vi "WF_Load_single_file_with_params.vi"(5 "Record#_START":i32, 8 "N of Record":i32, 9 "Record# STOP":i32, 10 "Enable limit = True":bool, 11 "WF_FILE_IN":path) -> (1 "Sampling rate":dbl, 2 "Record#":i32, 3 "Waveform":waveform(dbl), 4 "File_duration(s)":dbl)   [LabVIEW 2017]
uses:
  <vilib>/Waveform/WDTFileIO.llb/Read Waveform from File.vi
  <vilib>/Waveform/WDTOps.llb/WDT Append Waveforms DBL.vi
panel:
  out "Waveform Graph":waveform(dbl)(graph)
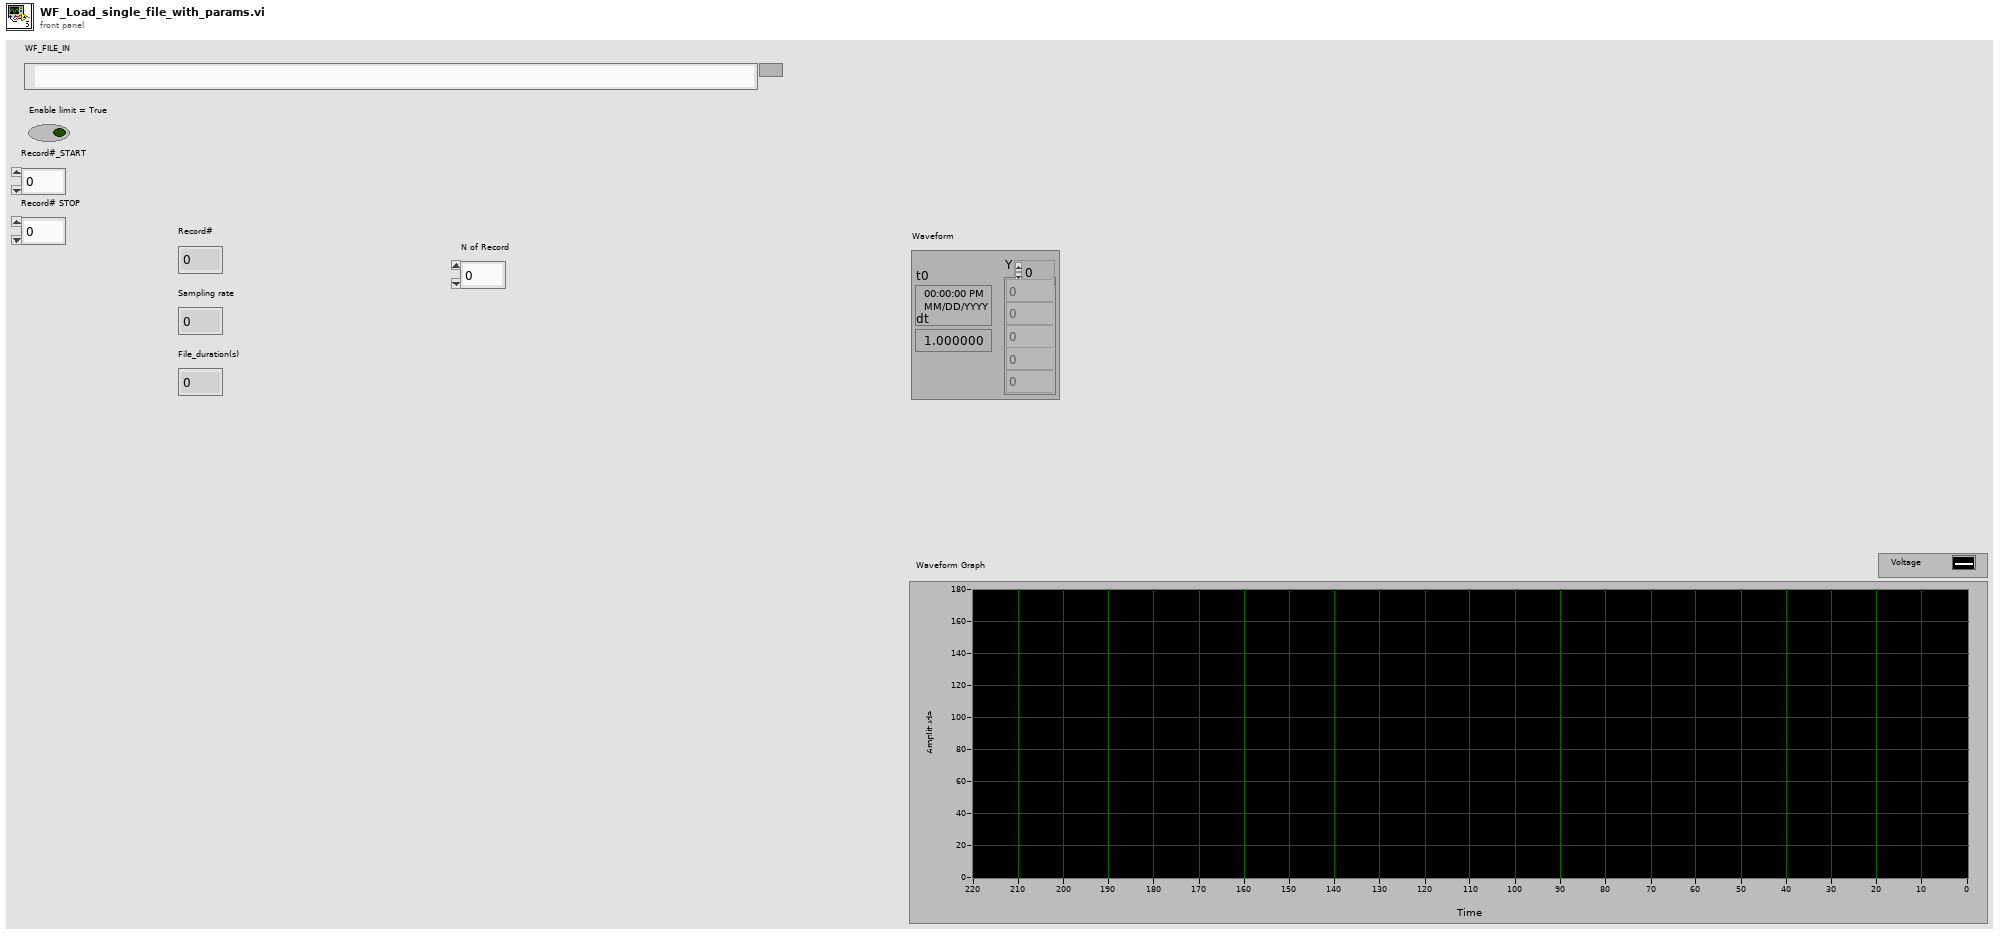
[diagram p1: front panel]
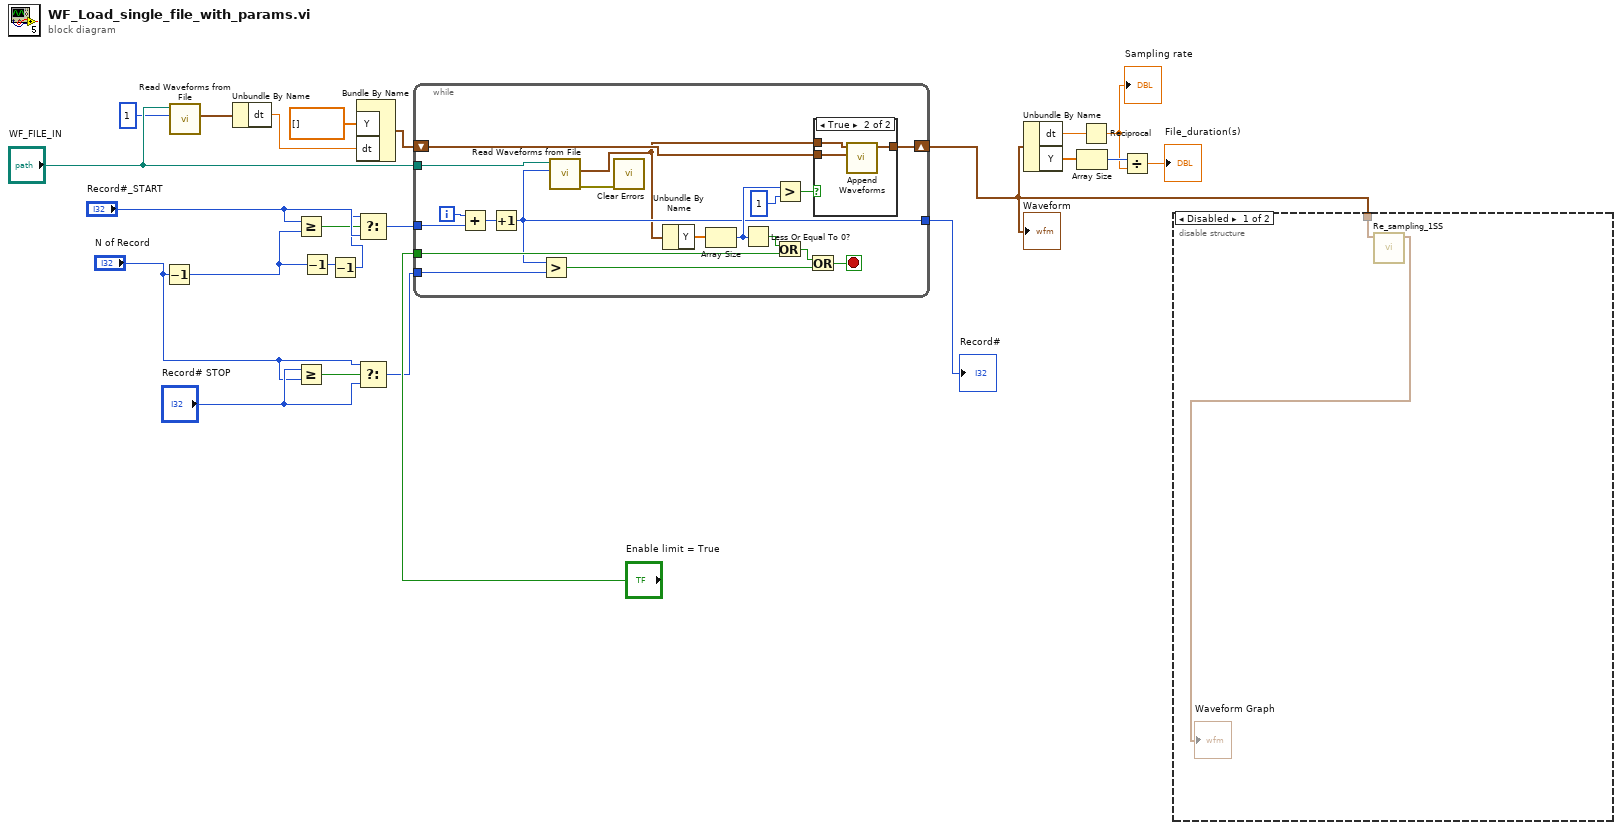
[diagram p0: block diagram]
diagram:
  n1 = Decrement(x="N of Record") -> (x-1=w5:i32)
  n2 = call-poly <vilib>:"Read Waveforms from File.vi"("offset (records:0)"=1, "file path (dialog if empty)"="WF_FILE_IN") -> ("first waveform in record"=w13:waveform(dbl))  [unwired: 4 in, 3 out]
  n3 = Unbundle By Name(w13) -> ("dt"=w16:dbl)
  n4 = Greater Or Equal?(x="Record#_START", y=w5) -> (x >= y?=w9:bool)
  n5 = Greater Or Equal?(x="Record# STOP", y="N of Record") -> (x >= y?=w7:bool)
  n6 = Decrement(x=w5) -> (x-1=w4:i32)
  n7 = Decrement(x=w4) -> (x-1=w3:i32)
  n8 = Bundle By Name("Y"=dbl[] [], "dt"=w16) -> (w17:waveform(dbl))  [unwired: 1 in]
  n9 = Select(t=w3, s=w9, f="Record#_START") -> (s? t:f=w10:i32)
  n10 = Select(t="N of Record", s=w7, f="Record# STOP") -> (s? t:f=w6:i32)
  n11 = while {
    shift-right: [w43] -> w1
    shift-left: w17 -> [w39]
    tunnel: "WF_FILE_IN" -> [w42]
    tunnel: "Enable limit = True" -> [w32]
    tunnel: [w30] -> w20
    tunnel: w10 -> [w31]
    tunnel: w6 -> [w29]
    i -> [w34]
    stop <- w26 stop-if-true
    n12 = Add(x=w34, y=w31) -> (x+y=w33:i32)
    n13 = Increment(x=w33) -> (x+1=w30:i32)
    n14 = Greater?(x=w30, y=w29) -> (0:w28:bool)
    n15 = call-poly <vilib>:"Read Waveforms from File.vi"("offset (records:0)"=w30, "file path (dialog if empty)"=w42) -> ("error out"=w40:errorcluster, "first waveform in record"=w25:waveform(dbl))  [unwired: 4 in, 2 out]
    n16 = call <vilib>:"Clear Errors.vi"("error in (no error)"=w40) -> ()  [unwired: 5 in, 2 out]
    n17 = Unbundle By Name(w25) -> ("Y"=w41:dbl[])
    n18 = Array Size(array=w41) -> (size(s)=w36:i32)
    n19 = Less Or Equal To 0?(x=w36) -> (x <= 0?=w35:bool)
    n20 = Greater?(x=w36, y=1) -> (0:w37:bool)
    n21 = Or(x=w35, y=w32) -> (x .or. y?=w27:bool)
    n22 = Or(x=w27, y=w28) -> (x .or. y?=w26:bool)
    n23 = case shown="True" w37 {
      tunnel: [w44 w47] -> w43
      tunnel: w25 -> [_ w45]
      tunnel: w39 -> [w44 w46]
      frame False {
      }
      frame True {
        n24 = call-poly <vilib>:"Append Waveforms.vi"("waveform B"=w46, "waveform A"=w45) -> ("waveform out"=w47:waveform(dbl))  [unwired: 8 in, 1 out]
      }
    }
  }
  "Record#" <- w20
  "Waveform" <- w1
  n25 = Unbundle By Name(w1) -> ("dt"=w21:dbl, "Y"=w22:dbl[])
  n26 = Array Size(array=w22) -> (size(s)=w23:i32)
  n27 = Reciprocal(x=w21) -> (1/x=w12:dbl)
  "Sampling rate" <- w12
  n28 = Divide(x=w23, y=w12) -> (x/y=→"File_duration(s)":dbl)
  n29 = disable-structure shown="Disabled" {
    disable-tunnel: w1 -> [w49 _]
    frame Disabled {
      n30 = call "Re_sampling_1SS.vi"("Waveform_main"=w49) -> ("Waveform"=→"Waveform Graph":waveform(dbl))  [unwired: 10 in]
    }
    frame Enabled {
    }
  }
